vi "DutyCycle.vi"(2 "AnalogTriggers":T1[](array[typedef])=[{"InHysteresis"=FALSE, "OverLimit"=FALSE, "Rising"=FALSE, "Falling"=FALSE}, {"InHysteresis"=FALSE, "OverLimit"=FALSE, "Rising"=FALSE, "Falling"=FALSE}, {"InHysteresis"=FALSE, "OverLimit"=FALSE, "Rising"=FALSE, "Falling"=FALSE}, {"InHysteresis"=FALSE, "OverLimit"=FALSE, "Rising"=FALSE, "Falling"=FALSE}, {"InHysteresis"=FALSE, "OverLimit"=FALSE, "Rising"=FALSE, "Falling"=FALSE}, {"InHysteresis"=FALSE, "OverLimit"=FALSE, "Rising"=FALSE, "Falling"=FALSE}, {"InHysteresis"=FALSE, "OverLimit"=FALSE, "Rising"=FALSE, "Falling"=FALSE}, {"InHysteresis"=FALSE, "OverLimit"=FALSE, "Rising"=FALSE, "Falling"=FALSE}], 3 "DigitalInputs":bool[](array[boolean])=[FALSE, FALSE, FALSE, FALSE, FALSE, FALSE, FALSE, FALSE, FALSE, FALSE, FALSE, FALSE, FALSE, FALSE, FALSE, FALSE, FALSE, FALSE, FALSE, FALSE, FALSE, FALSE, FALSE, FALSE, FALSE, FALSE, FALSE, FALSE, FALSE, FALSE, FALSE, FALSE], 4 "Source":T2) -> (0 "Frequency":fxp<+,11,11> format="%.21g", 1 "Output":fxp<+,31,31>)   [LabVIEW 2019]
uses:
  Helpers/Source.ctl
  Helpers/AnalogTriggerOutput.ctl
  <vilib>/rvi/Emulation/niFpgaProcessEmulError.vi
  <vilib>/rvi/Emulation/niFpgaSctlEmulationGetInTimedLoop.vi
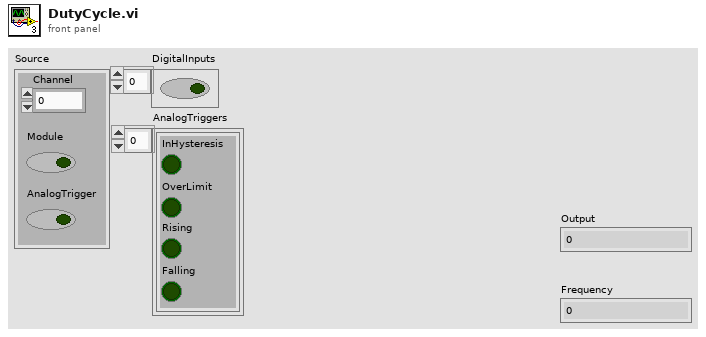
[diagram p1: front panel]
types:
  T1 = typedef "AnalogTriggerOutput.ctl" = cluster{"InHysteresis":bool, "OverLimit":bool, "Rising":bool, "Falling":bool}
  T2 = typedef "Source.ctl" = cluster{"Channel":fxp<+,4,4>, "Module":bool, "AnalogTrigger":bool}
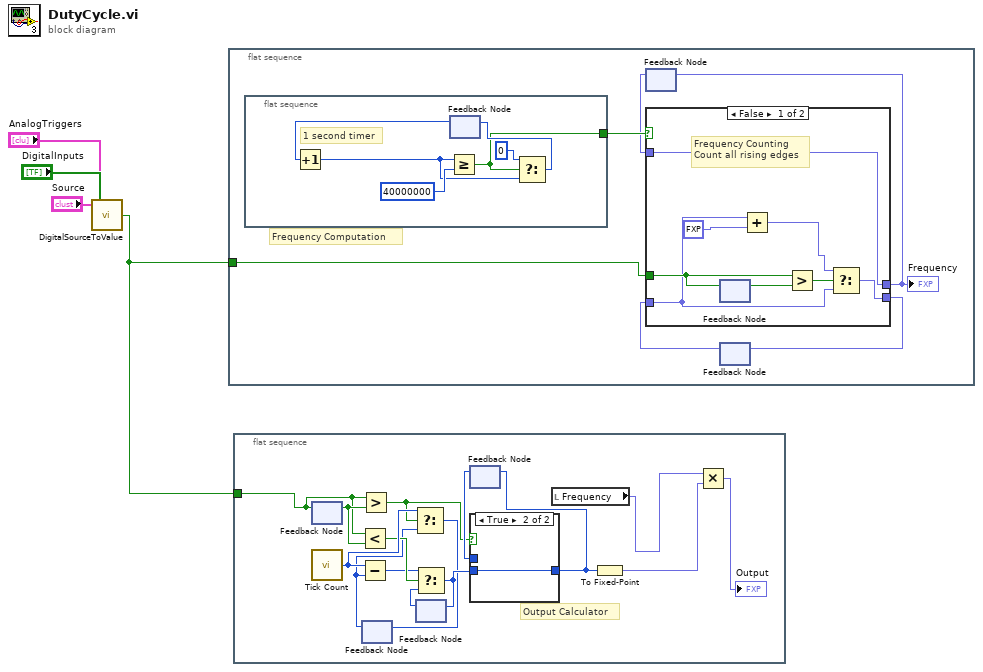
[diagram p0: block diagram]
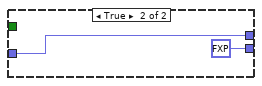
[diagram p3: hidden frame]
diagram:
  n1 = call "DigitalSourceToValue.vi"("AnalogTriggers"="AnalogTriggers", "DigitalInputs"="DigitalInputs", "Source"="Source") -> ("Value"=w1:bool)
  n2 = flat-sequence {
    tunnel: w1 -> [w5]
    frame #0 {
      # "Frequency Computation"
      n3 = flat-sequence {
        tunnel: [w21] -> w10
        frame #0 {
          # "1 second timer"
          n4 = feedback #1() -> (w23:u32)  [unwired: 1 in]
          n5 = Increment(x=w23) -> (x+1=w22:u32)
          n6 = Greater Or Equal?(x=w22, y=u32 40000000) -> (x >= y?=w21:bool)
          n7 = Select(t=u32 0, s=w21, f=w22) -> (s? t:f=w24:u32)
          n8 = feedback-in #1(w24) -> ()
        }
      }
      n9 = feedback #2() -> (w7:fxp<+,11,11>)  [unwired: 1 in]
      n10 = feedback #3() -> (w8:fxp<+,11,11>)  [unwired: 1 in]
      n11 = case shown="False" w10 {
        tunnel: w5 -> [w17 _]
        tunnel: [w15 fxp<+,11,11> 0.0] -> w9
        tunnel: w8 -> [w12 w19]
        tunnel: [w14 w19] -> w6
        tunnel: w7 -> [w14 _]
        frame False {
          # "Frequency Counting\nCount all rising edges"
          n12 = feedback #4() -> (w18:bool)  [unwired: 1 in]
          n13 = feedback-in #4(w17) -> ()
          n14 = Add(x=w12, y=fxp<+,11,11> 1.0) -> (x+y=w11:fxp<+,11,11>)
          n15 = Greater?(x=w17, y=w18) -> (0:w16:bool)
          n16 = Select(t=w11, s=w16, f=w12) -> (s? t:f=w15:fxp<+,11,11>)
        }
        frame True {
        }
      }
      "Frequency" <- w6
      n17 = feedback-in #2(w6) -> ()
      n18 = feedback-in #3(w9) -> ()
    }
  }
  n19 = flat-sequence {
    tunnel: w1 -> [w27]
    frame #0 {
      # "Output Calculator"
      n20 = feedback #5() -> (w38:bool)  [unwired: 1 in]
      n21 = feedback-in #5(w27) -> ()
      n22 = call "Tick Count"() -> ("Tick Count(Ticks)"=w41:u32)
      n23 = Less?(x=w27, y=w38) -> (x < y?=w40:bool)
      n24 = Greater?(x=w27, y=w38) -> (0:w36:bool)
      n25 = feedback #6() -> (w32:u32)  [unwired: 1 in]
      n26 = Subtract(x=w41, y=w32) -> (x-y=w37:u32)
      n27 = Select(t=w41, s=w36, f=w32) -> (s? t:f=w33:u32)
      n28 = feedback-in #6(w33) -> ()
      n29 = feedback #7() -> (w34:u32)  [unwired: 1 in]
      n30 = Select(t=w37, s=w40, f=w34) -> (s? t:f=w35:u32)
      n31 = feedback-in #7(w35) -> ()
      n32 = feedback #8() -> (w39:u32)  [unwired: 1 in]
      n33 = case shown="True" w36 {
        tunnel: w35 -> [_ w43]
        tunnel: [w42 w43] -> w31
        tunnel: w39 -> [w42 _]
        frame False {
        }
        frame True {
        }
      }
      n34 = feedback-in #8(w31) -> ()
      n35 = local read "Frequency"() -> (w30:fxp<+,11,11>)
      n36 = To Fixed-Point(number=w31) -> (fixed-point=w29:fxp<+,32,32>)  [unwired: 1 in]
      n37 = Multiply(x=w30, y=w29) -> (x*y=→"Output":fxp<+,31,31>)
    }
  }
